vi "TestExec.Control, Start Test.vi"(7 "Module Q Name":string, 8 "error in":errorcluster, 9 "Position":string, 10 "SN":string, 11 "Q In":refnum<queue>) -> (0 "error out":errorcluster)   [LabVIEW 2019]
uses:
  <vilib>/KATE/Queues/Q.Element.ctl
  <vilib>/KATE/Queues/Queue Utils.lvlib
panel:
  out "Q Out":refnum<queue>
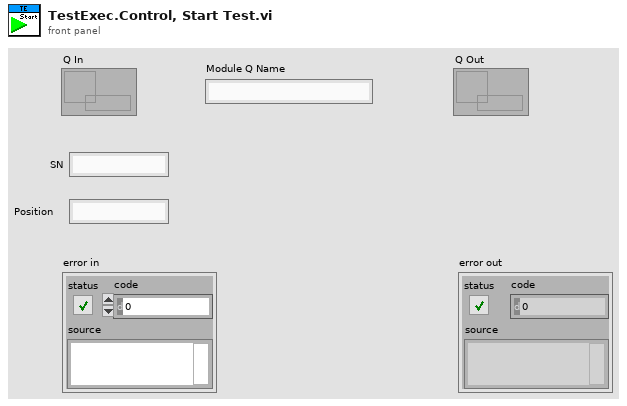
[diagram p1: front panel]
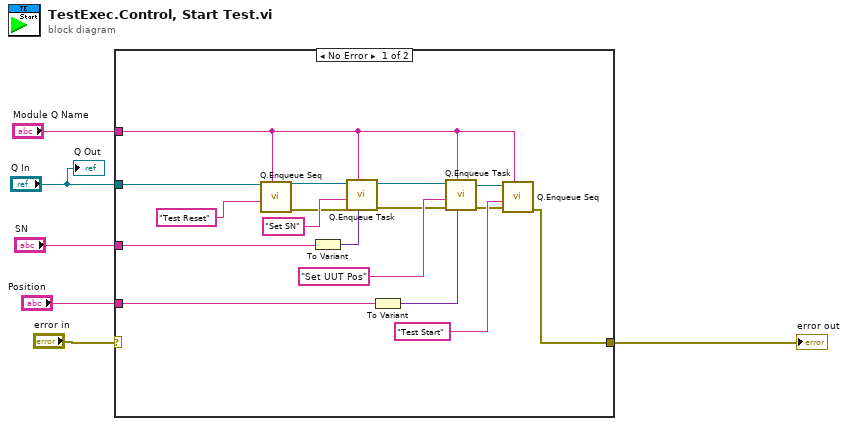
[diagram p0: block diagram]
diagram:
  n1 = case shown="No Error" "error in" {
    selector: "error in" -> [_ w24]
    tunnel: [w9 w24] -> w5
    tunnel: "Q In" -> [w14 _]
    tunnel: "Module Q Name" -> [w13 _]
    tunnel: "SN" -> [w8 _]
    tunnel: "Position" -> [w7 _]
    frame No Error {
      n2 = call <vilib>:"Q.Enqueue Seq.vi"("Q Name"=w13, "Seq Task Name"="Test Reset" ("Task Name"), "Q In"=w14) -> ("error out"=w12:errorcluster, "Q Out"=w16:refnum<queue>)  [unwired: 7 in]
      n3 = To Variant(anything=w8) -> (Variant=w21:variant)
      n4 = call <vilib>:"Q.Enqueue Task.vi"("Data1"=w21, "Q Name"=w13, "Error In"=w12, "Task Name"="Set SN", "Q In"=w16) -> ("error out"=w11:errorcluster, "Q Out"=w17:refnum<queue>)  [unwired: 5 in]
      n5 = To Variant(anything=w7) -> (Variant=w19:variant)
      n6 = call <vilib>:"Q.Enqueue Task.vi"("Data1"=w19, "Q Name"=w13, "Error In"=w11, "Task Name"="Set UUT Pos", "Q In"=w17) -> ("error out"=w10:errorcluster, "Q Out"=w15:refnum<queue>)  [unwired: 5 in]
      n7 = call <vilib>:"Q.Enqueue Seq.vi"("Q Name"=w13, "Error In"=w10, "Seq Task Name"="Test Start", "Q In"=w15) -> ("error out"=w9:errorcluster)  [unwired: 6 in, 1 out]
    }
    frame Error {
    }
  }
  "error out" <- w5
  "Q Out" <- "Q In"
